vi "CompleteTest.vi"() -> ()   [LabVIEW 2018]
uses:
  <vilib>/Studica/Studica Toolkit/Background/PWM Channel.ctl
  <vilib>/Studica/Studica Toolkit/Background/DIO Channel.ctl
  <vilib>/myRIO/Common/Instrument Driver Framework/myRIO v1.0/AI/typedefs/AI Channels List.ctl
  <vilib>/myRIO/Common/Instrument Driver Framework/myRIO v1.0/AI/typedefs/AI Channels Enum.ctl
  <vilib>/Studica/Studica Toolkit/Background/Mxp Selection.ctl
  <vilib>/Studica/Studica Toolkit/Background/I2C Channel.ctl
  <vilib>/Studica/Studica Toolkit/NavX/NavX.lvlib
panel:
  in  "Position A Servo 1":dbl(slide) scale=-200.0..200.0
  out "Sharp IR Distance 4":dbl
  out "Sharp IR Distance 3":dbl
  out "Sharp IR Distance 2":dbl
  out "Limit Switch":bool
  in  "Position B Servo 3":dbl(slide) scale=-200.0..200.0
  in  "Position B Servo 2":dbl(slide) scale=-200.0..200.0
  in  "Position B Servo 1":dbl(slide) scale=-200.0..200.0
  in  "Position A Servo 3":dbl(slide) scale=-200.0..200.0
  in  "Position A Servo 2":dbl(slide) scale=-200.0..200.0
  out "Ping A Inches":fxp<+,64,16>
  out "Ping A cm":fxp<+,64,16>
  out "Ping B Inches":fxp<+,64,16>
  out "Ping B cm":fxp<+,64,16>
  out "Left IR Sensor":dbl
  out "Distance M1 (inches) B":dbl
  out "Distance M0 (inches) B":dbl
  in  "Reset Encoder 3":bool
  in  "Reset Encoder 2":bool
  in  "Invert M1 B":bool
  in  "Invert M0 B":bool
  in  "Speed M1 B":dbl(slide) scale=-1.0..1.0
  in  "Speed M0 B":dbl(slide) scale=-1.0..1.0
  out "Distance M0 (inches)":dbl
  out "Distance M1 (inches)":dbl
  in  "Reset Encoder 1":bool
  in  "Reset Encoder 0":bool
  in  "Wheel Diameter (inches)":dbl format="%#_13g"
  in  "Ticks Per Rev":u32
  in  "stop":bool
  out "LSB Data":T1
  in  "Thresholds":dbl[](array[numeric])
  in  "Invert M1":bool
  in  "Speed M1":dbl(slide) scale=-1.0..1.0
  in  "Invert M0":bool
  in  "Speed M0":dbl(slide) scale=-1.0..1.0
  out "YRPHfH":T2
  out "Timestamp":u32
  in  "Zero Yaw":bool
  # "Set the encoder ticks \nand wheel diameter here\nfor acurate distance"
  # "Motors will only stop when \na value of 0 is applied"
  # "MXP B"
  # "MXP A"
  # "Press here to Zero the yaw"
  # "If stop is hit, motors will stop\nand robot will have to be reset\nbefore normal operation can \ncontinue."
  # "Set the LSB\nthresholds here\na value in the middle \nis best. Range (0-5)"
  # "MXP A\nPWM 3"
  # "MXP A\nPWM 4"
  # "MXP B\nPWM 3"
  # "MXP A\nPWM 2"
  # "MXP B\nPWM 2"
  # "MXP B\nPWM 3"
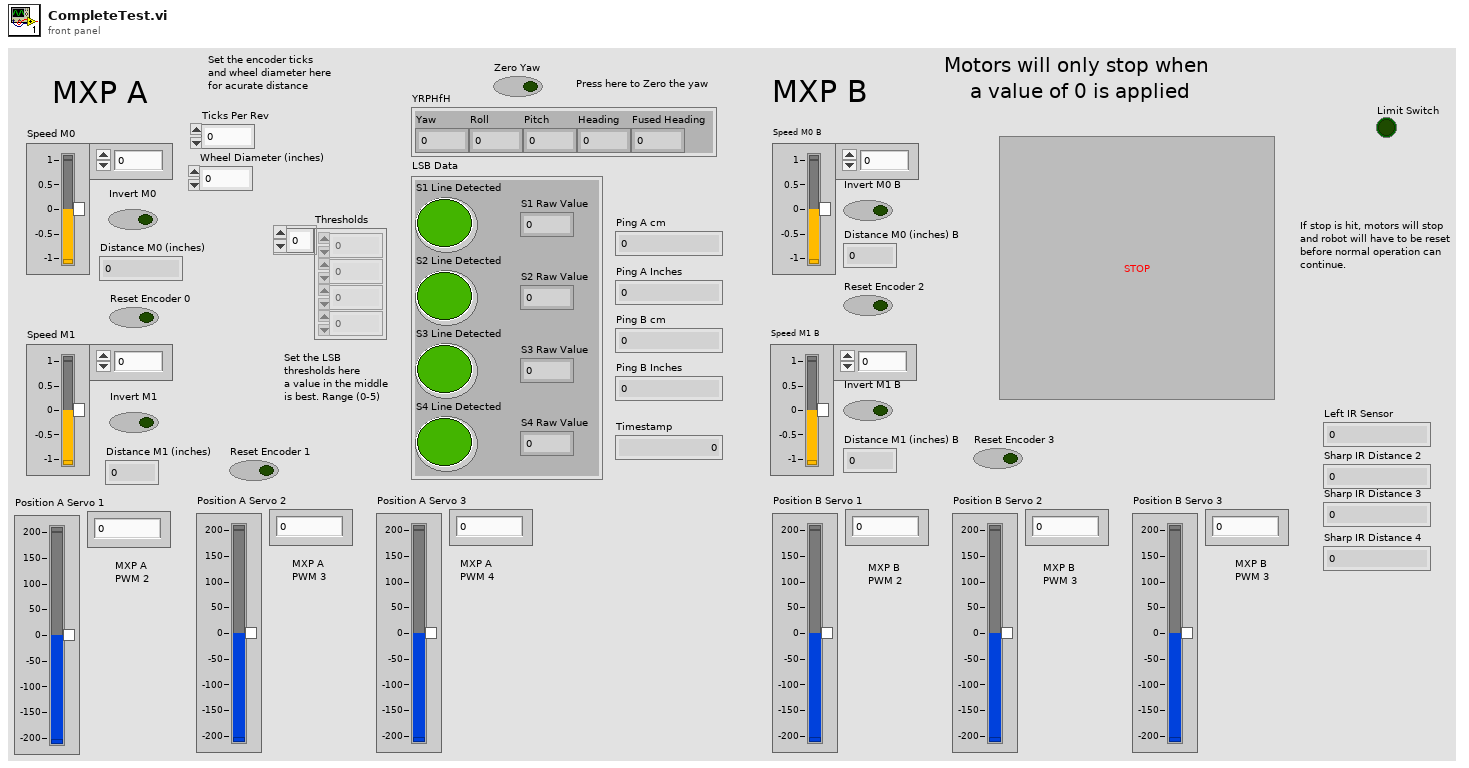
[diagram p1: front panel]
types:
  T1 = cluster{"S1 Line Detected":bool, "S2 Line Detected":bool, "S3 Line Detected":bool, "S4 Line Detected":bool, "S1 Raw Value":dbl, "S2 Raw Value":dbl, "S3 Raw Value":dbl, "S4 Raw Value":dbl}
  T2 = cluster{"Yaw":dbl, "Roll":dbl, "Pitch":dbl, "Heading":dbl, "Fused Heading":dbl}
  T3 = typedef "DIO Channel.ctl" = enum16{"Not Connected", "A/DIO1", "A/DIO2", "A/DIO3", "A/DIO4", "A/DIO5", "A/DIO6", "A/DIO7", "A/DIO13", "B/DIO1", "B/DIO2", "B/DIO3", "B/DIO4", "B/DIO5", "B/DIO6", "B/DIO7", "B/DIO13", "C/DIO0", "C/DIO1", "C/DIO2", "C/DIO3", "C/DIO4", "C/DIO5", "C/DIO6", "C/DIO7"}
  T4 = typedef "PWM Channel.ctl" = enum16{"Not Connected", "A/PWM0", "A/PWM1", "A/PWM2", "A/PWM3", "A/PWM4", "B/PWM0", "B/PWM1", "B/PWM2", "B/PWM3", "B/PWM4", "C/PWM0", "C/PWM1"}
  T5 = typedef "Mxp Selection.ctl" = enum16{"MXP A", "MXP B"}
  T6 = typedef "I2C Channel.ctl" = enum16{"Not Connected", "A", "B"}
  T7 = cluster{"I2C Ref Out":cluster{"I2C Channel":T6, "FPGA VI Reference Out":refnum<k20>}, "Connected":bool, "Slave Address (7-bit)":u8, "Registry":u8[]}
  T8 = cluster{"DIO Channel":T3, "FPGA VI Reference Out":refnum<k20>}
  T9 = cluster{"PWM Channel":T4, "FPGA VI Reference Out":refnum<k20>}
  T10 = typedef "AI Channels List.ctl" = T11[]
  T11 = typedef "AI Channels Enum.ctl" = enum16{"Not Connected", "AudioIn/Left", "AudioIn/Right", "C/AI0", "C/AI1", "A/AI0", "A/AI1", "A/AI2", "A/AI3", "A/AI4", "A/AI5", "A/AI6", "A/AI7", "B/AI0", "B/AI1", "B/AI2", "B/AI3", "B/AI4", "B/AI5", "B/AI6", "B/AI7", "AI/AI0", "AI/AI1", "AI/AI2", "AI/AI3", "A/AI0 (DIFF)", "A/AI1 (DIFF)", "A/AI2 (DIFF)", "A/AI3 (DIFF)", "B/AI0 (DIFF)", "B/AI1 (DIFF)", "B/AI2 (DIFF)", "B/AI3 (DIFF)"}
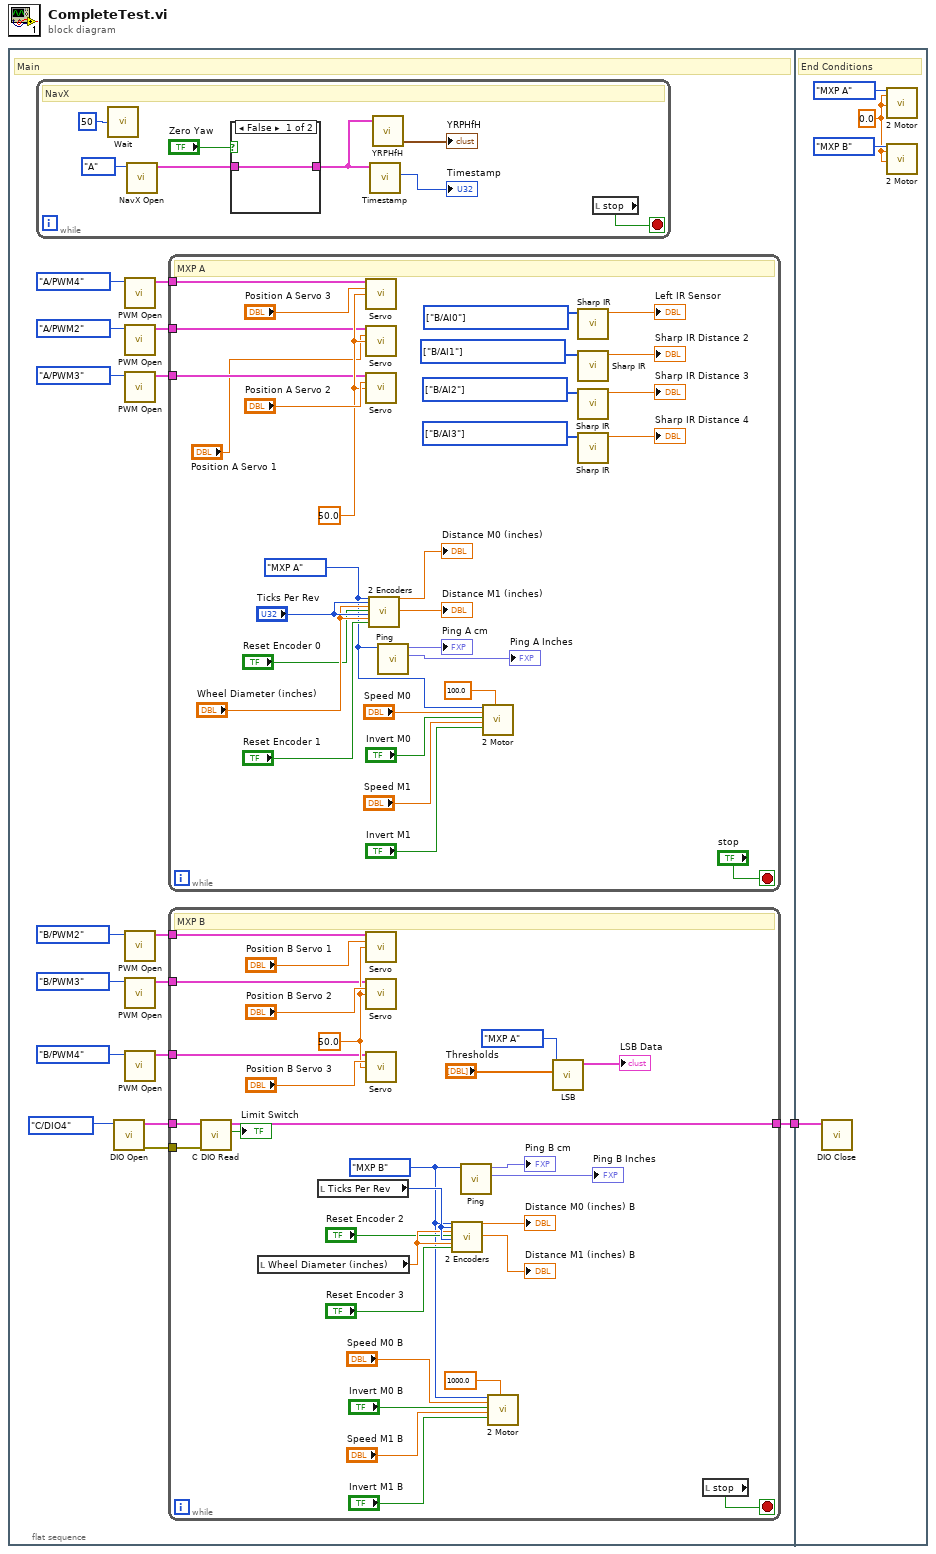
[diagram p0: block diagram]
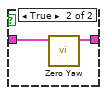
[diagram p2: hidden frame]
diagram:
  n1 = flat-sequence {
    tunnel: [w4] -> w1
    tunnel: w1 -> [w88]
    frame #0 {
      # "Main"
      n2 = while {
        stop <- w47 stop-if-true
        # "NavX"
        n3 = call "Wait"("Count(mSec)"=u32 50) -> ()  [unwired: 1 out]
        n4 = call <vilib>:"NavX Open.vi"("I2C Channel"=I2C_Channel."A") -> ("NavX Info"=w51:T7)  [unwired: 9 in, 1 out]
        n5 = case shown="False" "Zero Yaw" {
          tunnel: w51 -> [w55 w57]
          tunnel: [w55 w56] -> w52
          frame False {
          }
          frame True {
            n6 = call <vilib>:"Zero Yaw.vi"("NavX Info In"=w57) -> ("NavX Info Out"=w56:T7)  [unwired: 10 in]
          }
        }
        n7 = call <vilib>:"Timestamp.vi"("NavX Info In"=w52) -> ("Timestamp"=→"Timestamp":u32)  [unwired: 9 in, 1 out]
        n8 = call <vilib>:"YRPHfH.vi"("NavX Info In"=w52) -> ("YRPHfH"=→"YRPHfH":T2)  [unwired: 3 in, 1 out]
        n9 = local read "stop"() -> (w47:bool)
      }
      n10 = call <vilib>:"DIO Open.vi"("DIO Channel"=DIO_Channel."C/DIO4") -> ("error out"=w3:errorcluster, "DIO Info Out"=w5:T8)  [unwired: 9 in]
      n11 = call <vilib>:"PWM Open.vi"("PWM Channel"=PWM_Channel."A/PWM4") -> ("PWM Info Out"=w14:T9)  [unwired: 9 in, 1 out]
      n12 = call <vilib>:"PWM Open.vi"("PWM Channel"=PWM_Channel."A/PWM2") -> ("PWM Info Out"=w12:T9)  [unwired: 9 in, 1 out]
      n13 = call <vilib>:"PWM Open.vi"("PWM Channel"=PWM_Channel."A/PWM3") -> ("PWM Info Out"=w13:T9)  [unwired: 9 in, 1 out]
      n14 = call <vilib>:"PWM Open.vi"("PWM Channel"=PWM_Channel."B/PWM2") -> ("PWM Info Out"=w8:T9)  [unwired: 9 in, 1 out]
      n15 = call <vilib>:"PWM Open.vi"("PWM Channel"=PWM_Channel."B/PWM3") -> ("PWM Info Out"=w7:T9)  [unwired: 9 in, 1 out]
      n16 = call <vilib>:"PWM Open.vi"("PWM Channel"=PWM_Channel."B/PWM4") -> ("PWM Info Out"=w6:T9)  [unwired: 9 in, 1 out]
      n17 = while {
        tunnel: w14 -> [w70]
        tunnel: w13 -> [w69]
        tunnel: w12 -> [w68]
        stop <- "stop" stop-if-true
        w60 = T10 [enum."B/AI3"] items=["Not Connected", "AudioIn/Left", "AudioIn/Right", "C/AI0", "C/AI1", "A/AI0", "A/AI1", "A/AI2", "A/AI3", "A/AI4", "A/AI5", "A/AI6", "A/AI7", "B/AI0", "B/AI1", "B/AI2", "B/AI3", "B/AI4", "B/AI5", "B/AI6", "B/AI7", "AI/AI0", "AI/AI1", "AI/AI2", "AI/AI3", "A/AI0 (DIFF)", "A/AI1 (DIFF)", "A/AI2 (DIFF)", "A/AI3 (DIFF)", "B/AI0 (DIFF)", "B/AI1 (DIFF)", "B/AI2 (DIFF)", "B/AI3 (DIFF)"] ("AI Channel 3")
        w61 = T10 [enum."B/AI2"] items=["Not Connected", "AudioIn/Left", "AudioIn/Right", "C/AI0", "C/AI1", "A/AI0", "A/AI1", "A/AI2", "A/AI3", "A/AI4", "A/AI5", "A/AI6", "A/AI7", "B/AI0", "B/AI1", "B/AI2", "B/AI3", "B/AI4", "B/AI5", "B/AI6", "B/AI7", "AI/AI0", "AI/AI1", "AI/AI2", "AI/AI3", "A/AI0 (DIFF)", "A/AI1 (DIFF)", "A/AI2 (DIFF)", "A/AI3 (DIFF)", "B/AI0 (DIFF)", "B/AI1 (DIFF)", "B/AI2 (DIFF)", "B/AI3 (DIFF)"] ("AI Channel 3")
        w64 = T10 [enum."B/AI1"] items=["Not Connected", "AudioIn/Left", "AudioIn/Right", "C/AI0", "C/AI1", "A/AI0", "A/AI1", "A/AI2", "A/AI3", "A/AI4", "A/AI5", "A/AI6", "A/AI7", "B/AI0", "B/AI1", "B/AI2", "B/AI3", "B/AI4", "B/AI5", "B/AI6", "B/AI7", "AI/AI0", "AI/AI1", "AI/AI2", "AI/AI3", "A/AI0 (DIFF)", "A/AI1 (DIFF)", "A/AI2 (DIFF)", "A/AI3 (DIFF)", "B/AI0 (DIFF)", "B/AI1 (DIFF)", "B/AI2 (DIFF)", "B/AI3 (DIFF)"] ("AI Channel 2")
        w65 = T10 [enum."B/AI0"] items=["Not Connected", "AudioIn/Left", "AudioIn/Right", "C/AI0", "C/AI1", "A/AI0", "A/AI1", "A/AI2", "A/AI3", "A/AI4", "A/AI5", "A/AI6", "A/AI7", "B/AI0", "B/AI1", "B/AI2", "B/AI3", "B/AI4", "B/AI5", "B/AI6", "B/AI7", "AI/AI0", "AI/AI1", "AI/AI2", "AI/AI3", "A/AI0 (DIFF)", "A/AI1 (DIFF)", "A/AI2 (DIFF)", "A/AI3 (DIFF)", "B/AI0 (DIFF)", "B/AI1 (DIFF)", "B/AI2 (DIFF)", "B/AI3 (DIFF)"] ("AI Channel")
        w71 = 50.0
        w76 = Mxp_Selection."MXP A" ("Mxp Side")
        # "MXP A"
        n18 = call <vilib>:"Servo.vi"("PWM Info In"=w70, "Position"="Position A Servo 3", "Frequency [Hz]"=w71) -> ()  [unwired: 11 in, 2 out]
        n19 = call <vilib>:"Servo.vi"("PWM Info In"=w68, "Position"="Position A Servo 1", "Frequency [Hz]"=w71) -> ()  [unwired: 11 in, 2 out]
        n20 = call <vilib>:"Servo.vi"("PWM Info In"=w69, "Position"="Position A Servo 2", "Frequency [Hz]"=w71) -> ()  [unwired: 11 in, 2 out]
        n21 = call <vilib>:"2 Encoders.vi"("Mxp Side"=w76, "Ticks Per Rev M0"="Ticks Per Rev", "Wheel Diameter M0 (inches)"="Wheel Diameter (inches)", "Reset Encoder 0"="Reset Encoder 0", "Ticks Per Rev M1"="Ticks Per Rev", "Wheel Diameter M1 (inches)"="Wheel Diameter (inches)", "Reset Encoder 1"="Reset Encoder 1") -> ("Distance M0 (inches)"=→"Distance M0 (inches)":dbl, "Distance M1 (inches)"=→"Distance M1 (inches)":dbl)  [unwired: 18 in, 1 out]
        n22 = call <vilib>:"Ping.vi"("Mxp Side"=w76) -> ("IN"=→"Ping A Inches":fxp<+,64,16>, "CM"=→"Ping A cm":fxp<+,64,16>)  [unwired: 8 in, 1 out]
        n23 = call <vilib>:"2 Motor.vi"("Mxp Side"=w76, "Speed M0"="Speed M0", "Invert M0"="Invert M0", "Speed M1"="Speed M1", "Invert M1"="Invert M1", "Frequency [Hz]"=100.0) -> ()  [unwired: 13 in, 1 out]
        n24 = call <vilib>:"Sharp IR.vi"("AI Channel"=w65) -> ("Sharp IR Distance"=→"Left IR Sensor":dbl)  [unwired: 8 in, 2 out]
        n25 = call <vilib>:"Sharp IR.vi"("AI Channel"=w64) -> ("Sharp IR Distance"=→"Sharp IR Distance 2":dbl)  [unwired: 8 in, 2 out]
        n26 = call <vilib>:"Sharp IR.vi"("AI Channel"=w61) -> ("Sharp IR Distance"=→"Sharp IR Distance 3":dbl)  [unwired: 8 in, 2 out]
        n27 = call <vilib>:"Sharp IR.vi"("AI Channel"=w60) -> ("Sharp IR Distance"=→"Sharp IR Distance 4":dbl)  [unwired: 8 in, 2 out]
      }
      n28 = while {
        tunnel: w8 -> [w27]
        tunnel: w7 -> [w26]
        tunnel: w6 -> [w25]
        tunnel: w5 -> [w21]
        tunnel: [w20] -> w4
        tunnel: w3 -> [w18]
        stop <- w46 stop-if-true
        w28 = 50.0
        w34 = Mxp_Selection."MXP B" ("Mxp Side")
        # "MXP B"
        n29 = call <vilib>:"C DIO Read.vi"("error in (no error)"=w18, "DIO Info In in"=w21) -> ("IN"=→"Limit Switch":bool, "DIO Info In out"=w20:T8)  [unwired: 7 in, 1 out]
        n30 = local read "Wheel Diameter (inches)"() -> (w39:dbl)
        n31 = local read "Ticks Per Rev"() -> (w40:u32)
        n32 = call <vilib>:"Servo.vi"("PWM Info In"=w27, "Position"="Position B Servo 1", "Frequency [Hz]"=w28) -> ()  [unwired: 11 in, 2 out]
        n33 = call <vilib>:"Servo.vi"("PWM Info In"=w26, "Position"="Position B Servo 2", "Frequency [Hz]"=w28) -> ()  [unwired: 11 in, 2 out]
        n34 = call <vilib>:"Servo.vi"("PWM Info In"=w25, "Position"="Position B Servo 3", "Frequency [Hz]"=w28) -> ()  [unwired: 11 in, 2 out]
        n35 = call <vilib>:"2 Encoders.vi"("Mxp Side"=w34, "Ticks Per Rev M0"=w40, "Wheel Diameter M0 (inches)"=w39, "Reset Encoder 0"="Reset Encoder 2", "Ticks Per Rev M1"=w40, "Wheel Diameter M1 (inches)"=w39, "Reset Encoder 1"="Reset Encoder 3") -> ("Distance M0 (inches)"=→"Distance M0 (inches) B":dbl, "Distance M1 (inches)"=→"Distance M1 (inches) B":dbl)  [unwired: 18 in, 1 out]
        n36 = call <vilib>:"Ping.vi"("Mxp Side"=w34) -> ("IN"=→"Ping B Inches":fxp<+,64,16>, "CM"=→"Ping B cm":fxp<+,64,16>)  [unwired: 8 in, 1 out]
        n37 = call <vilib>:"2 Motor.vi"("Mxp Side"=w34, "Speed M0"="Speed M0 B", "Invert M0"="Invert M0 B", "Speed M1"="Speed M1 B", "Invert M1"="Invert M1 B", "Frequency [Hz]"=1000.0) -> ()  [unwired: 13 in, 1 out]
        n38 = call <vilib>:"LSB.vi"("Thresholds"="Thresholds", "Mxp Side"=Mxp_Selection."MXP A") -> ("LSB Data"=→"LSB Data":T1)  [unwired: 8 in, 1 out]
        n39 = local read "stop"() -> (w46:bool)
      }
    }
    frame #1 {
      w89 = 0.0
      # "End Conditions"
      n40 = call <vilib>:"DIO Close.vi"("DIO Info In"=w88) -> ()  [unwired: 10 in, 1 out]
      n41 = call <vilib>:"2 Motor.vi"("Mxp Side"=Mxp_Selection."MXP A", "Speed M0"=w89, "Speed M1"=w89) -> ()  [unwired: 16 in, 1 out]
      n42 = call <vilib>:"2 Motor.vi"("Mxp Side"=Mxp_Selection."MXP B", "Speed M0"=w89, "Speed M1"=w89) -> ()  [unwired: 16 in, 1 out]
    }
  }
